vi "Terminal-Main-LubricateUnit.vi"(4 "ErrorQRef":refnum<queue>, 5 "ModbusNResRef":refnum<notifier>, 6 "ModbusMsgQRef":refnum<queue>, 7 "ModbusNReqRef":refnum<notifier>, 8 "error in (no error)":errorcluster caption="错误输入（无错误）", 11 "LubricateUnitNRef":refnum<notifier>) -> (0 "error out":errorcluster caption="错误输出")   [LabVIEW 2014]
panel:
  out "Lubricate Unit is running":bool
  out "LubricateUnit开始通知器":refnum<notifier>
  out "LubricateUnit开始响应器":refnum<notifier>
  out "LubricateUnit停止通知器":refnum<notifier>
  out "LubricateUnit停止响应器":refnum<notifier>
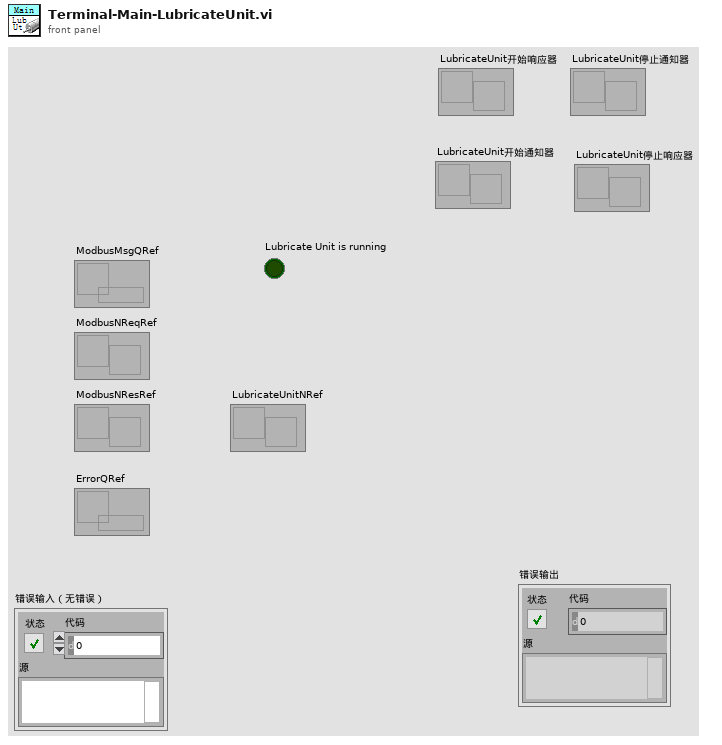
[diagram p1: front panel]
types:
  T1 = cluster{"Transaction ID":u16, "Unit ID":u8, "Starting Address":u16, "Quantity":u16}
  T2 = cluster{"switch":bool, "L":u16, "T":u16, "P":u16}
  T3 = cluster{"Transaction ID":u16, "Unit ID":u8, "Address":u16, "Register":u16}
  T4 = cluster{"Transaction ID":u16, "Unit ID":u8, "Starting Address":u16, "Registers":u16[]}
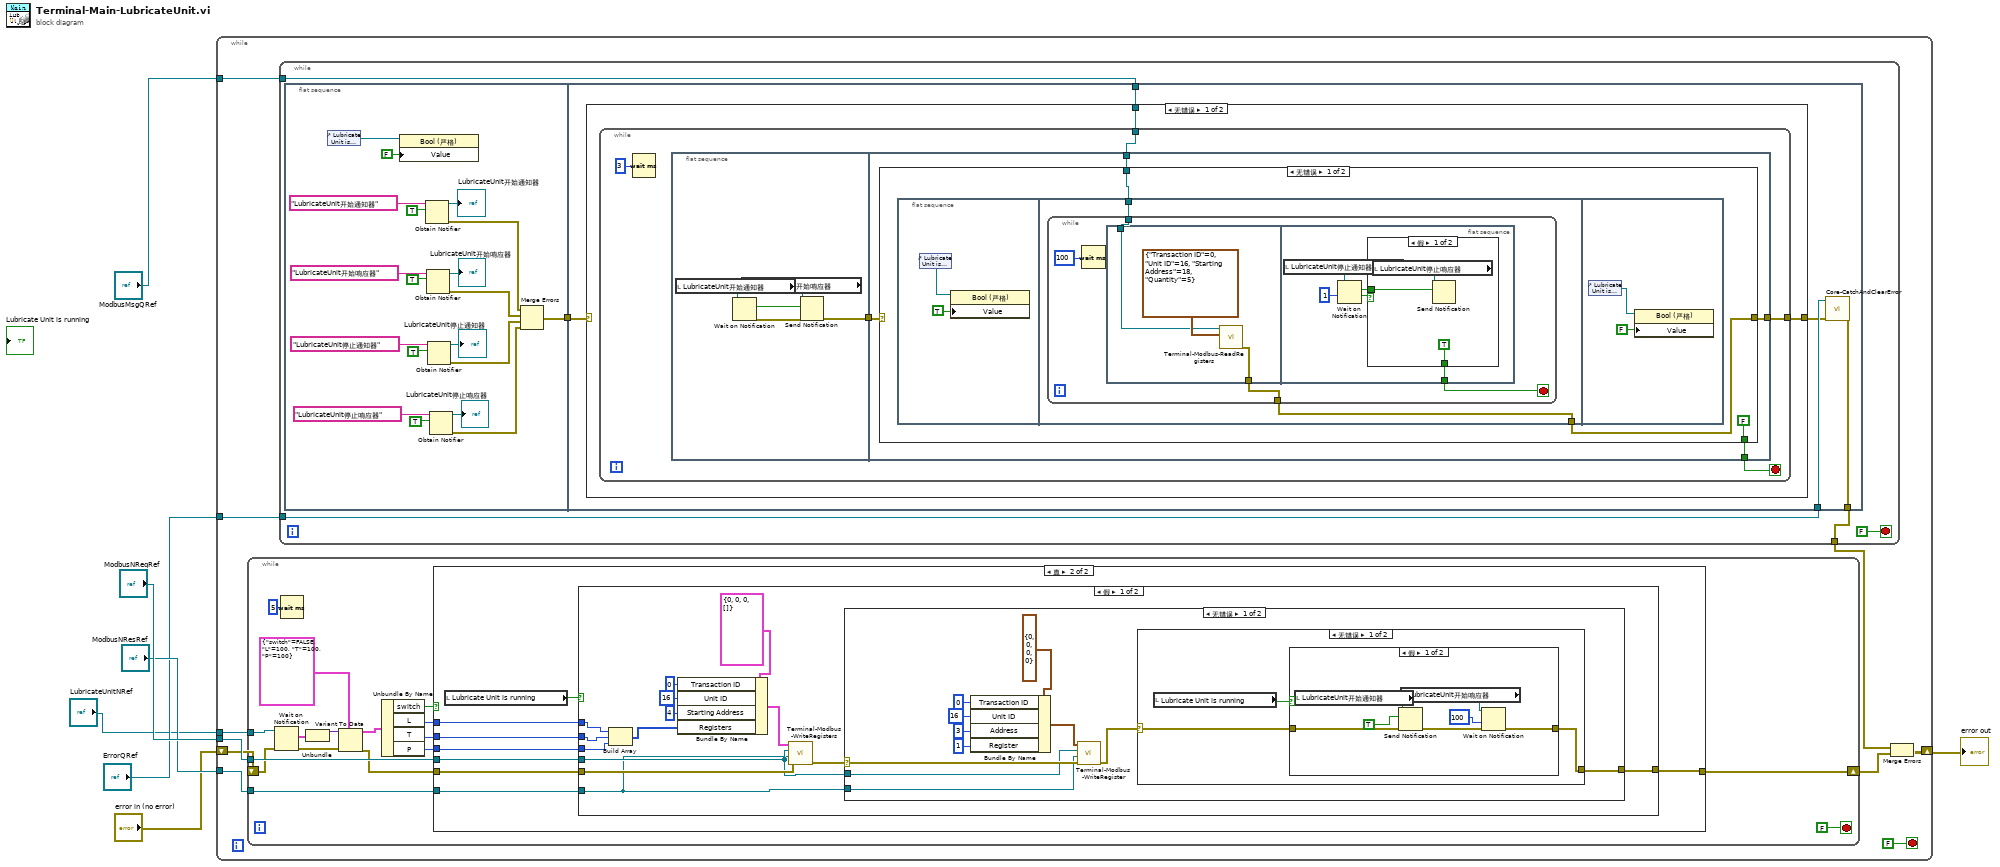
[diagram p0: block diagram]
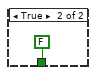
[diagram p2: hidden frame]
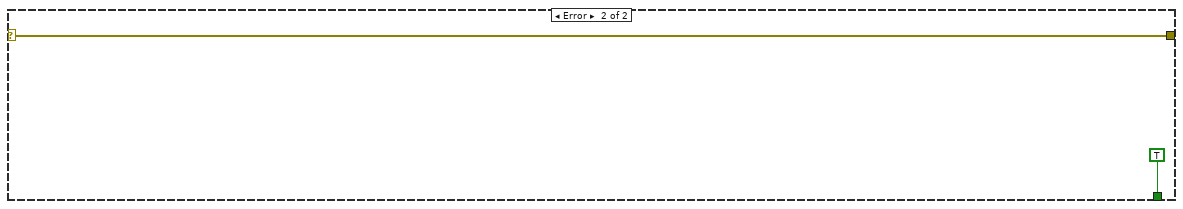
[diagram p3: hidden frame]
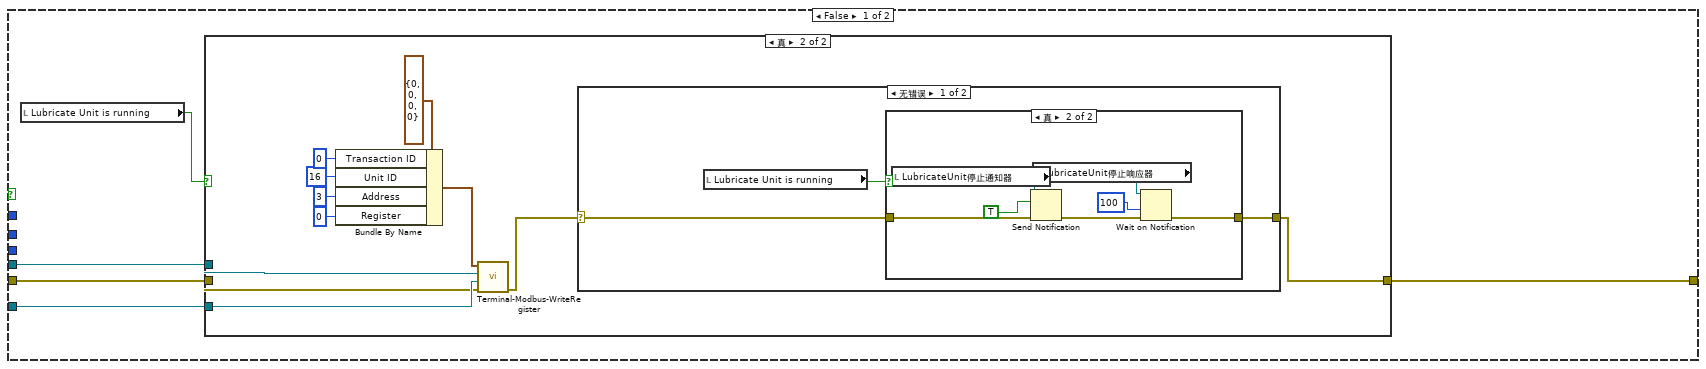
[diagram p5: hidden frame]
diagram:
  n1 = while {
    tunnel: "ModbusMsgQRef" -> [w17]
    tunnel: "ModbusNReqRef" -> [w16]
    tunnel: "ModbusNResRef" -> [w15]
    tunnel: "ErrorQRef" -> [w13]
    shift-right: [w12] -> w2
    shift-left: "error in (no error)" -> [w14]
    tunnel: "LubricateUnitNRef" -> [w8]
    stop <- FALSE stop-if-true
    n2 = while {
      tunnel: w16 -> [w107]
      tunnel: w15 -> [w106]
      shift-right: [w105] -> w11
      shift-left: w14 -> [w101]
      tunnel: w8 -> [w102]
      stop <- FALSE stop-if-true
      n3 = Wait on Notification(notifier=w102, error in (no error)=w101) -> (notification=w100:cluster{variant, string}, error out=w95:errorcluster)  [unwired: 2 in, 2 out]
      n4 = Wait (ms)(milliseconds to wait=u32 5 ("等待时间（毫秒）")) -> ()  [unwired: 1 out]
      n5 = Unbundle(w100) -> (w99:variant)  [unwired: 1 out]
      n6 = Variant To Data(error in=w95, type=T2 {"switch"=FALSE, "L"=100, "T"=100, "P"=100}, Variant=w99) -> (data=w98:T2, error out=w94:errorcluster)
      n7 = Unbundle By Name(w98) -> ("switch"=w97:bool, "L"=w96:u16, "T"=w92:u16, "P"=w91:u16)
      n8 = case shown="真" w97 {
        tunnel: w107 -> [w112 w142]
        tunnel: w106 -> [w111 w143]
        tunnel: w94 -> [w110 w144]
        tunnel: [w109 w141] -> w105
        tunnel: w96 -> [_ w140]
        tunnel: w92 -> [_ w138]
        tunnel: w91 -> [_ w137]
        frame False {
          n9 = local read "Lubricate Unit is running"() -> (w108:bool)
          n10 = case shown="真" w108 {
            tunnel: w112 -> [_ w123]
            tunnel: w111 -> [_ w122]
            tunnel: w110 -> [w113 w121]
            tunnel: [w113 w120] -> w109
            frame False {
            }
            frame True {
              n11 = Bundle By Name(cluster=T3 {"Transaction ID"=0, "Unit ID"=0, "Address"=0, "Register"=0} ("簇"), "Transaction ID"=u16 0, "Unit ID"=u8 16, "Address"=u16 3, "Register"=u16 0) -> (w115:T3)
              n12 = call "Terminal-Modbus-WriteRegister.vi"("error in (no error)"=w121, "ModbusNResRef"=w122, "ModbusNReqRef"=w123, "簇"=w115) -> ("error out"=w124:errorcluster)  [unwired: 7 in]
              n13 = case shown="无错误" w124 {
                selector: w124 -> [w126 w136]
                tunnel: [w125 w136] -> w120
                frame No Error {
                  n14 = local read "Lubricate Unit is running"() -> (w127:bool)
                  n15 = case shown="真" w127 {
                    tunnel: [w128 w130] -> w125
                    tunnel: w126 -> [w128 w129]
                    frame False {
                    }
                    frame True {
                      n16 = local read "LubricateUnit停止通知器"() -> (w135:refnum<notifier>)
                      n17 = Send Notification(notification=TRUE ("通知"), notifier=w135, error in (no error)=w129) -> (error out=w133:errorcluster)  [unwired: 1 out]
                      n18 = local read "LubricateUnit停止响应器"() -> (w132:refnum<notifier>)
                      n19 = Wait on Notification(notifier=w132, timeout in ms (-1)=100 ("超时毫秒(-1)"), error in (no error)=w133) -> (error out=w130:errorcluster)  [unwired: 1 in, 3 out]
                    }
                  }
                }
                frame Error {
                }
              }
            }
          }
        }
        frame True {
          n20 = local read "Lubricate Unit is running"() -> (w139:bool)
          n21 = case shown="假" w139 {
            tunnel: w144 -> [w157 w183]
            tunnel: w143 -> [w145 _]
            tunnel: w142 -> [w146 _]
            tunnel: [w156 w183] -> w141
            tunnel: w140 -> [w155 _]
            tunnel: w138 -> [w154 _]
            tunnel: w137 -> [w153 _]
            frame False {
              n22 = Build Array(w155, w154, w153) -> (w147:u16[])
              n23 = Bundle By Name(cluster=T4 {"Transaction ID"=0, "Unit ID"=0, "Starting Address"=0, "Registers"=[]} ("簇"), "Transaction ID"=u16 0, "Unit ID"=u8 16, "Starting Address"=u16 4 ("Address"), "Registers"=w147) -> (w149:T4)
              n24 = call "Terminal-Modbus-WriteRegisters.vi"("error in (no error)"=w157, "ModbusNResRef"=w145, "ModbusNReqRef"=w146, "簇"=w149) -> ("error out"=w158:errorcluster)  [unwired: 7 in]
              n25 = case shown="无错误" w158 {
                selector: w158 -> [w168 w182]
                tunnel: w146 -> [w167 _]
                tunnel: w145 -> [w166 _]
                tunnel: [w165 w182] -> w156
                frame No Error {
                  n26 = Bundle By Name(cluster=T3 {"Transaction ID"=0, "Unit ID"=0, "Address"=0, "Register"=0} ("簇"), "Transaction ID"=u16 0, "Unit ID"=u8 16, "Address"=u16 3, "Register"=u16 1) -> (w160:T3)
                  n27 = call "Terminal-Modbus-WriteRegister.vi"("error in (no error)"=w168, "ModbusNResRef"=w166, "ModbusNReqRef"=w167, "簇"=w160) -> ("error out"=w169:errorcluster)  [unwired: 7 in]
                  n28 = case shown="无错误" w169 {
                    selector: w169 -> [w171 w181]
                    tunnel: [w170 w181] -> w165
                    frame No Error {
                      n29 = local read "Lubricate Unit is running"() -> (w172:bool)
                      n30 = case shown="假" w172 {
                        tunnel: [w174 w180] -> w170
                        tunnel: w171 -> [w173 w180]
                        frame False {
                          n31 = local read "LubricateUnit开始通知器"() -> (w179:refnum<notifier>)
                          n32 = Send Notification(notification=TRUE ("通知"), notifier=w179, error in (no error)=w173) -> (error out=w177:errorcluster)  [unwired: 1 out]
                          n33 = local read "LubricateUnit开始响应器"() -> (w176:refnum<notifier>)
                          n34 = Wait on Notification(notifier=w176, timeout in ms (-1)=100 ("超时毫秒(-1)"), error in (no error)=w177) -> (error out=w174:errorcluster)  [unwired: 1 in, 3 out]
                        }
                        frame True {
                        }
                      }
                    }
                    frame Error {
                    }
                  }
                }
                frame Error {
                }
              }
            }
            frame True {
            }
          }
        }
      }
    }
    n35 = while {
      tunnel: w17 -> [w21]
      tunnel: w13 -> [w20]
      tunnel: [w18] -> w10
      stop <- FALSE stop-if-true
      n36 = flat-sequence {
        tunnel: [w24] -> w22
        tunnel: w22 -> [w46]
        tunnel: w20 -> [w45]
        tunnel: [w43] -> w18
        tunnel: w21 -> [w42]
        frame #0 {
          n37 = control-ref of="Lubricate Unit is running"() -> (w23:refnum<vi>)
          n38 = property class="Bool (严格)"(reference=w23, "Value"=FALSE ("值")) -> ()  [unwired: 1 in, 2 out]
          n39 = Obtain Notifier(name (unnamed)="LubricateUnit开始通知器" ("名称（未命名）"), notification data type=TRUE) -> (notifier out=→"LubricateUnit开始通知器":refnum<notifier>, error out=w28:errorcluster)  [unwired: 2 in, 1 out]
          n40 = Obtain Notifier(name (unnamed)="LubricateUnit开始响应器" ("名称（未命名）"), notification data type=TRUE) -> (notifier out=→"LubricateUnit开始响应器":refnum<notifier>, error out=w27:errorcluster)  [unwired: 2 in, 1 out]
          n41 = Obtain Notifier(name (unnamed)="LubricateUnit停止通知器" ("名称（未命名）"), notification data type=TRUE) -> (notifier out=→"LubricateUnit停止通知器":refnum<notifier>, error out=w26:errorcluster)  [unwired: 2 in, 1 out]
          n42 = Obtain Notifier(name (unnamed)="LubricateUnit停止响应器" ("名称（未命名）"), notification data type=TRUE) -> (notifier out=→"LubricateUnit停止响应器":refnum<notifier>, error out=w25:errorcluster)  [unwired: 2 in, 1 out]
          n43 = Merge Errors(w28, w27, w26, w25) -> (w24:errorcluster)
        }
        frame #1 {
          n44 = case shown="无错误" w46 {
            selector: w46 -> [_ w90]
            tunnel: [w48 w90] -> w44
            tunnel: w42 -> [w47 _]
            frame No Error {
              n45 = while {
                tunnel: [w51] -> w48
                tunnel: w47 -> [w50]
                stop <- w52 stop-if-true
                n46 = Wait (ms)(milliseconds to wait=u32 3 ("等待时间（毫秒）")) -> ()  [unwired: 1 out]
                n47 = flat-sequence {
                  tunnel: [w54] -> w53
                  tunnel: w53 -> [w62]
                  tunnel: [w61] -> w52
                  tunnel: [w60] -> w51
                  tunnel: w50 -> [w59]
                  frame #0 {
                    n48 = local read "LubricateUnit开始通知器"() -> (w58:refnum<notifier>)
                    n49 = Wait on Notification(notifier=w58) -> (notification=w55:bool, error out=w56:errorcluster)  [unwired: 3 in, 2 out]
                    n50 = local read "LubricateUnit开始响应器"() -> (w57:refnum<notifier>)
                    n51 = Send Notification(notification=w55, notifier=w57, error in (no error)=w56) -> (error out=w54:errorcluster)  [unwired: 1 out]
                  }
                  frame #1 {
                    n52 = case shown="无错误" w62 {
                      selector: w62 -> [_ w88]
                      tunnel: [FALSE TRUE] -> w61
                      tunnel: [w64 w88] -> w60
                      tunnel: w59 -> [w63 _]
                      frame No Error {
                        n53 = flat-sequence {
                          tunnel: [w68] -> w64
                          tunnel: w63 -> [w69]
                          frame #0 {
                            n54 = control-ref of="Lubricate Unit is running"() -> (w66:refnum<vi>)
                            n55 = property class="Bool (严格)"(reference=w66, "Value"=TRUE ("值")) -> ()  [unwired: 1 in, 2 out]
                          }
                          frame #1 {
                            n56 = while {
                              tunnel: w69 -> [w73]
                              tunnel: [w72] -> w68
                              stop <- w71 stop-if-true
                              n57 = Wait (ms)(milliseconds to wait=u32 100 ("等待时间（毫秒）")) -> ()  [unwired: 1 out]
                              n58 = flat-sequence {
                                tunnel: w73 -> [w75]
                                tunnel: [w74] -> w72
                                tunnel: [w77] -> w71
                                frame #0 {
                                n59 = call "Terminal-Modbus-ReadRegisters.vi"("簇"=T1 {"Transaction ID"=0, "Unit ID"=16, "Starting Address"=18, "Quantity"=5}, "ModbusMsgQRef"=w75) -> ("error out"=w74:errorcluster)  [unwired: 9 in]
                                }
                                frame #1 {
                                n60 = local read "LubricateUnit停止通知器"() -> (w80:refnum<notifier>)
                                n61 = Wait on Notification(notifier=w80, timeout in ms (-1)=1 ("超时毫秒(-1)")) -> (notification=w78:bool, timed out?=w79:bool)  [unwired: 2 in, 2 out]
                                n62 = case shown="假" w79 {
                                tunnel: [TRUE FALSE] -> w77
                                tunnel: w78 -> [w83 _]
                                frame False {
                                n63 = local read "LubricateUnit停止响应器"() -> (w82:refnum<notifier>)
                                n64 = Send Notification(notification=w83, notifier=w82) -> ()  [unwired: 1 in, 2 out]
                                }
                                frame True {
                                }
                                }
                                }
                              }
                            }
                          }
                          frame #2 {
                            n65 = control-ref of="Lubricate Unit is running"() -> (w86:refnum<vi>)
                            n66 = property class="Bool (严格)"(reference=w86, "Value"=FALSE ("值")) -> ()  [unwired: 1 in, 2 out]
                          }
                        }
                      }
                      frame Error {
                      }
                    }
                  }
                }
              }
            }
            frame Error {
            }
          }
          n67 = call "Core-CatchAndClearError.vi"("error in (no error)"=w44, "ErrorQ"=w45) -> ("error out"=w43:errorcluster)  [unwired: 7 in]
        }
      }
    }
    n68 = Merge Errors(w10, w11) -> (w12:errorcluster)
  }
  "error out" <- w2
